vi "Measurement Logic.vi"() -> ()   [LabVIEW 2020, in "CancellableMeasurement.lvlib"]
uses:
  CancellableMeasurement.lvlib
  Measurement Configuration.ctl
  Measurement Results.ctl
  <vilib>/MeasurementLink/MeasurementLink Measurement Server/Classes/MeasurementContext/MeasurementContext.lvclass
  <vilib>/MeasurementLink/MeasurementLink Measurement Server/Classes/MeasurementContext/Accessor/Is Canceled.vi
panel:
  out "Measurement Context out":refnum<class "MeasurementContext.lvclass">
  in  "Measurement Context":refnum<class "MeasurementContext.lvclass">
  out "Measurement Results":T1
  in  "Measurement Configuration":T2={"delay"=10.0}
  out "error out":errorcluster
  in  "error in":errorcluster
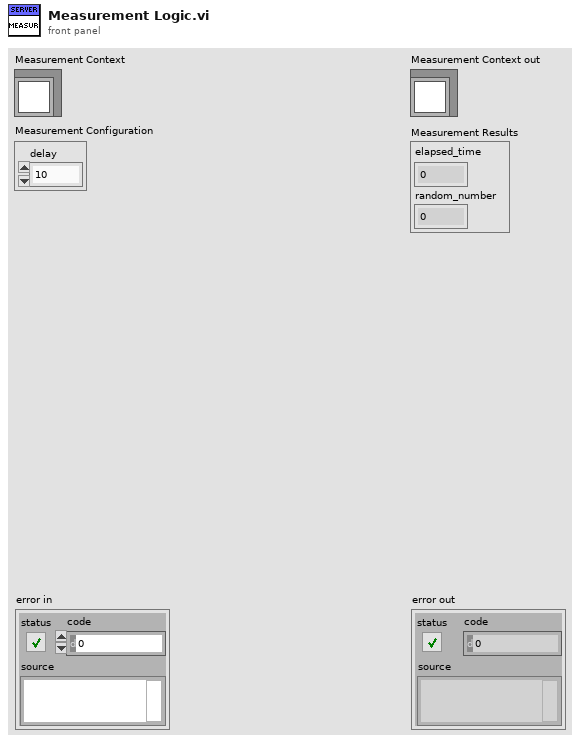
[diagram p1: front panel]
types:
  T1 = typedef "CancellableMeasurement.lvlib/Measurement Results.ctl" = cluster{"elapsed_time":dbl, "random_number":dbl}
  T2 = typedef "CancellableMeasurement.lvlib/Measurement Configuration.ctl" = cluster{"delay":dbl}
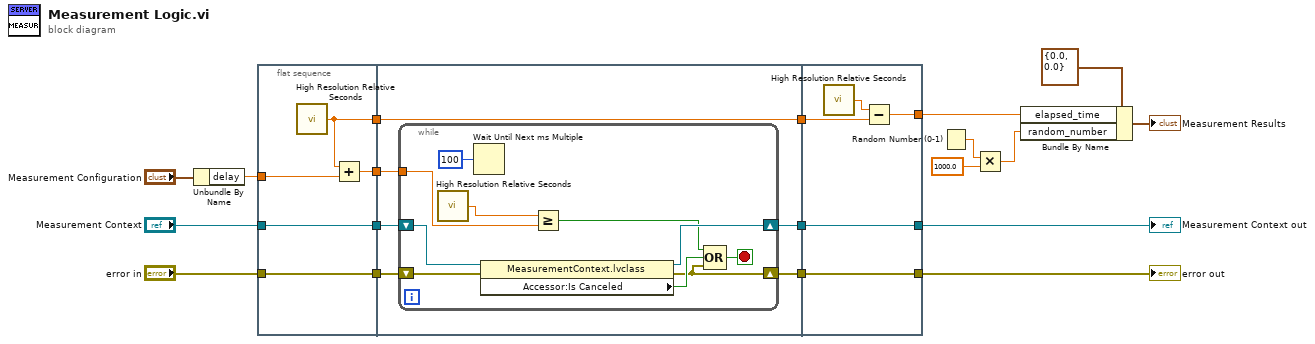
[diagram p0: block diagram]
diagram:
  n1 = Unbundle By Name("Measurement Configuration") -> ("delay"=w7:dbl)
  n2 = flat-sequence {
    tunnel: "error in" -> [w23]
    tunnel: "Measurement Context" -> [w24]
    tunnel: [w24] -> w19
    tunnel: [w23] -> w18
    tunnel: [w22] -> w17
    tunnel: [w21] -> w16
    tunnel: w7 -> [w20]
    tunnel: [w29] -> w15
    tunnel: [w26] -> w14
    tunnel: [w25] -> w13
    tunnel: w19 -> [w30]
    tunnel: w18 -> [w28]
    tunnel: w17 -> [w27]
    tunnel: w16 -> [w25]
    tunnel: [w45] -> w9
    tunnel: w15 -> [w45]
    tunnel: w14 -> [w42]
    tunnel: w13 -> [w43]
    tunnel: [w41] -> w5
    tunnel: [w42] -> w10
    frame #0 {
      n3 = call <vilib>:"High Resolution Relative Seconds.vi"() -> ("relative seconds"=w21:dbl)
      n4 = Add(x=w21, y=w20) -> (x+y=w22:dbl)
    }
    frame #1 {
      n5 = while {
        shift-right: [w36] -> w29
        shift-left: w30 -> [w39]
        shift-right: [w32] -> w26
        shift-left: w28 -> [w35]
        tunnel: w27 -> [w33]
        stop <- w38 stop-if-true
        n6 = call <vilib>:"High Resolution Relative Seconds.vi"() -> ("relative seconds"=w34:dbl)
        n7 = Wait Until Next ms Multiple(millisecond multiple=u32 100) -> ()  [unwired: 1 out]
        n8 = property class="MeasurementContext.lvclass"(reference=w39, error in=w35) -> (reference out=w36:refnum<class "MeasurementContext.lvclass">, error out=w32:errorcluster, "Accessor:Is Canceled"=w37:bool)
        n9 = Greater Or Equal?(x=w34, y=w33) -> (x >= y?=w31:bool)
        n10 = Compound Arithmetic op=OR(w31, w37, w32) -> (w38:bool)
      }
    }
    frame #2 {
      n11 = call <vilib>:"High Resolution Relative Seconds.vi"() -> ("relative seconds"=w44:dbl)
      n12 = Subtract(x=w44, y=w43) -> (x-y=w41:dbl)
    }
  }
  n13 = Random Number (0-1)() -> (number: 0 to 1=w4:dbl)
  n14 = Multiply(x=w4, y=1000.0) -> (x*y=w2:dbl)
  n15 = Bundle By Name(cluster=T1 {"elapsed_time"=0.0, "random_number"=0.0} ("Measurement Results"), "elapsed_time"=w5, "random_number"=w2) -> (→"Measurement Results":T1)
  "error out" <- w10
  "Measurement Context out" <- w9
